vi "Read.vi"(8 "error in (no error)":errorcluster, 11 "Numeric Command Config in":refnum<class "Numeric Command Config.lvclass">) -> (0 "error out":errorcluster, 1 "Command":dbl, 2 "Channel":string, 3 "Numeric Command Config out":refnum<class "Numeric Command Config.lvclass">)   [LabVIEW 2020, in "VolatusSeqConfig.lvlib" / "Numeric Command Config.lvclass"]
uses:
  Numeric Command Config.lvclass
  Numeric Command Config.lvclass/Numeric Command Config.ctl
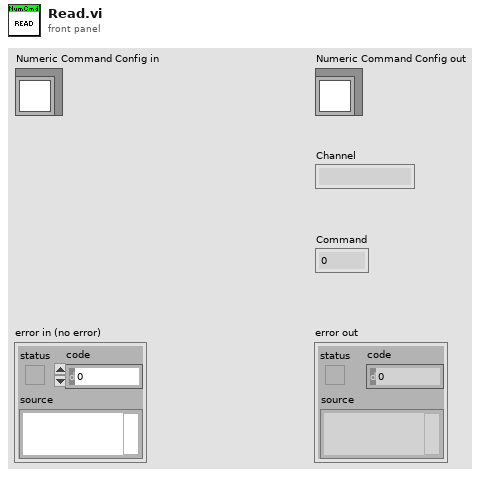
[diagram p1: front panel]
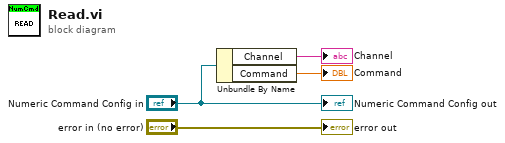
[diagram p0: block diagram]
diagram:
  n1 = Unbundle By Name("Numeric Command Config in") -> ("Channel"=→"Channel":string, "Command"=→"Command":dbl)
  "error out" <- "error in (no error)"
  "Numeric Command Config out" <- "Numeric Command Config in"
